vi "synnax writer write.vi"(8 "error in (no error)":errorcluster, 9 "data":dbl[](array[numeric])=array[4097 elements], 10 "channel":u32, 11 "writer":u64) -> (0 "error out":errorcluster, 3 "writer out":u64)   [LabVIEW 2026, in "synnax_clib.lvlib"]
doc: "SYNNAX_EXPORT int32_t synnax_writer_write(\n SynnaxWriter writer,\n uint32_t channel,\n const double *data,\n uint64_t sample_count,\n SynnaxError err\n);"
uses:
  synnax_clib.lvlib
  synnax_clib.dll
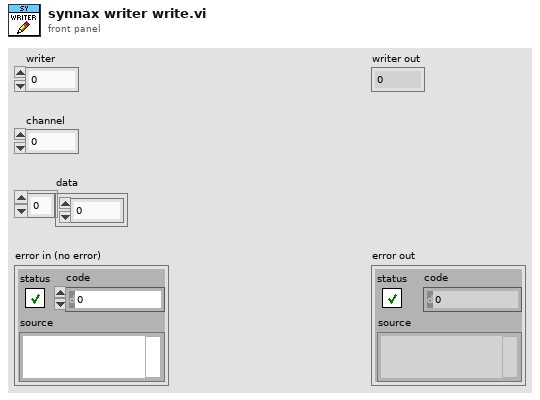
[diagram p1: front panel]
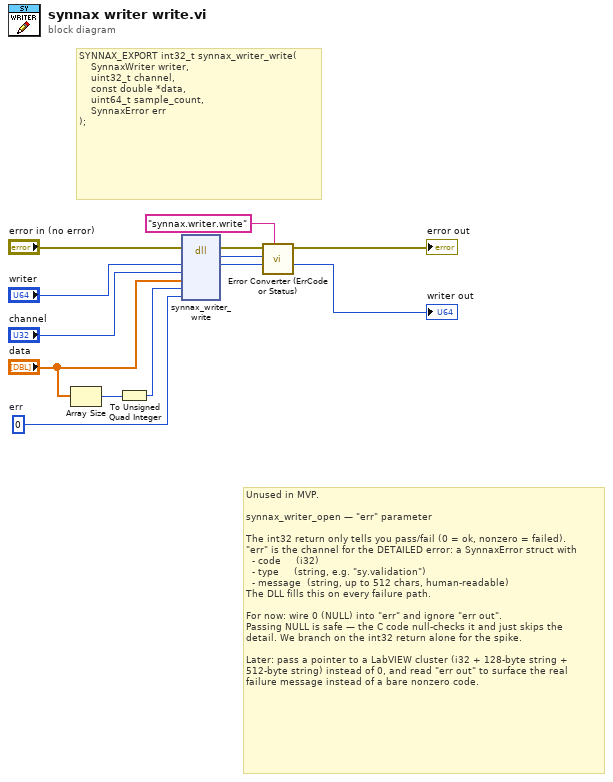
[diagram p0: block diagram]
diagram:
  w8 = u64 0  # err
  # "Unused in MVP.\n\nsynnax_writer_open — \"err\" parameter\n\nThe int32 return only tells you pass/fail (0 = ok, nonzero = failed).\n\"err\" is the channel for the DETAILED error: a SynnaxError struct with\n  - code     (i32)\n  - type     (string, e.g. \"sy.validation\")\n  - message  (string, up to 512 chars, human-readable)\nThe DLL fills this on every failure path.\n\nFor now: wire 0 (NULL) into \"err\" and ignore \"err out\".\nPassing NULL is safe — the C code null-checks it and just skips the\ndetail. We branch on the int32 return alone for the spike.\n\nLater: pass a pointer to a LabVIEW cluster (i32 + 128-byte string +\n512-byte string) instead of 0, and read \"err out\" to surface the real\nfailure message instead of a bare nonzero code."
  # "SYNNAX_EXPORT int32_t synnax_writer_write(\n    SynnaxWriter writer,\n    uint32_t channel,\n    const double *data,\n    uint64_t sample_count,\n    SynnaxError err\n);"
  n1 = Array Size(array="data") -> (size(s)=w6:i32)
  n2 = To Unsigned Quad Integer(1:w6) -> (0:w5:u64)
  n3 = dll-call lib="C/synnax/client/labview/lvlib/synnax_clib.*" fn="synnax_writer_write"(error in="error in (no error)", "writer"="writer", "channel"="channel", "data"="data", "sample_count"=w5, "err"=w8) -> (error out=w4:errorcluster, "return type"=w3:i32, "writer"=→"writer out":u64)  [unwired: 6 in, 1 out]
  n4 = call "Error Converter (ErrCode or Status).vi"("source"="synnax.writer.write", "error code"=w3, "error in (no error)"=w4) -> ("error out"=→"error out":errorcluster)  [unwired: 8 in]
